vi "Requests.vi"(8 "error in (no error)":errorcluster, 9 "write enable":bool=TRUE, 11 "ICPCON ET7024 in":refnum<class "ICPCON ET-7024AO.lvclass">) -> (0 "error out":errorcluster, 3 "ICPCON ET7024 out":refnum<class "ICPCON ET-7024AO.lvclass">)   [LabVIEW 2021, in "ICPCON ET-7024AO.lvclass"]
uses:
  ICPCON ET-7024AO.lvclass
  D:/my_projects/projects/21/Master CR/Master CR.lvclass
  D:/my_projects/projects/21/Master CR/Devices/ET7000/TCP/TCP.lvclass
  Master CR.lvclass/Master CR.ctl
  Modbus_v121c/Modbus Data Unit/Modbus Data Unit.lvclass/Modbus Data Unit.ctl
  Modbus_v121c/Network Protocol/Network Master/Network Master.lvclass/Network Master.ctl
  Network Protocol/Read Network Protocol.vi
  Modbus_v121c/Master Function Definition/Write Multiple Registers Request.vi
  Modbus_v121c/Master Function Definition/Function data mismatch error.vi
  Modbus_v121c/Master Function Definition/Write Multiple Registers Response.vi
  Modbus_v121c/Network Protocol/Network Master/Read write Master.vi
  Modbus_v121c/Master Function Definition/Read Holding Registers Request.vi
  Modbus_v121c/Master Function Definition/Read Holding Registers Response.vi
  Modbus_v121c/Modbus Data Unit/Construct PDU.vi
  Modbus_v121c/Utility/U16s to Bytes.vi
  Modbus_v121c/Master Function Definition/Function code mismatch error.vi
  Modbus_v121c/Data Model/Error Generator.vi
  Modbus_v121c/Modbus Data Unit/Deconstruct PDU.vi
  Modbus_v121c/Utility/Bytes to U16s.vi
  TCP/TCP.lvclass
  Modbus_v121c/Network Protocol/Network Master/Network Master.lvclass
  Modbus_v121c/Modbus Data Unit/Modbus Data Unit.lvclass
  Modbus_v121c/Data Model/Device Data Model.lvclass
  Modbus_v121c/Transmission Data Unit/Transmission Data Unit.lvclass
  Master CR.lvclass
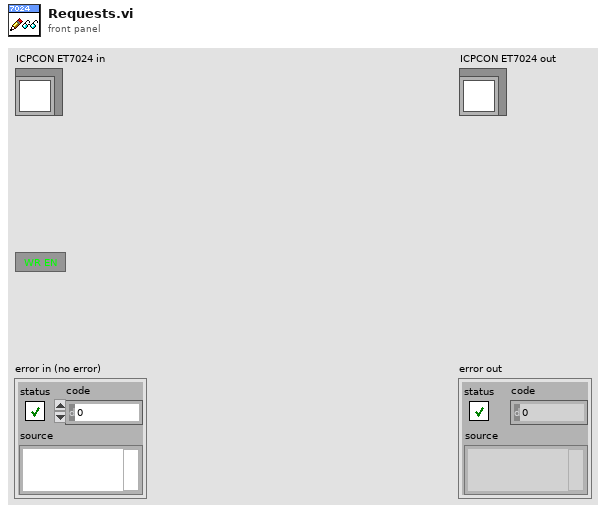
[diagram p1: front panel]
types:
  T1 = typedef "Device Data Model.lvclass/N channel.ctl" = cluster{"N DI channel":i32, "N DO channel":i32, "N AI channel":i32, "N AO channel":i32}
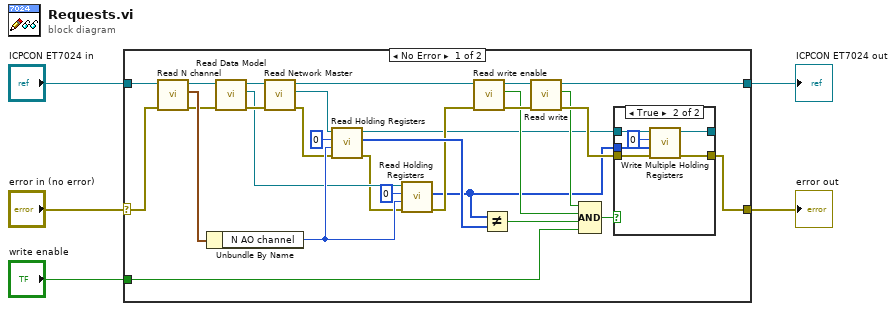
[diagram p0: block diagram]
diagram:
  n1 = case shown="No Error" "error in (no error)" {
    selector: "error in (no error)" -> [w31 w44]
    tunnel: [w27 w44] -> w3
    tunnel: [w26 w43] -> w4
    tunnel: "ICPCON ET7024 in" -> [w33 w43]
    tunnel: "write enable" -> [w28 _]
    frame No Error {
      n2 = call "Read N channel.vi"("error in (no error)"=w31, "Master CR in"=w33) -> ("error out"=w30:errorcluster, "N channel"=w34:T1, "Master CR out"=w32:refnum<class "ICPCON ET-7024AO.lvclass">)  [unwired: 7 in]
      n3 = Unbundle By Name(w34) -> ("N AO channel"=w29:i32)
      n4 = call "Read Data Model.vi"("error in (no error)"=w30, "Master CR in"=w32) -> ("error out"=w24:errorcluster, "Data Model"=w20:refnum<class "Device Data Model.lvclass">, "Master CR out"=w25:refnum<class "ICPCON ET-7024AO.lvclass">)  [unwired: 7 in]
      n5 = call "Read Network Master.vi"("error in (no error)"=w24, "TCP in"=w25) -> ("error out"=w21:errorcluster, "Network Master"=w22:refnum<class "Network Master.lvclass">, "TCP out"=w23:refnum<class "ICPCON ET-7024AO.lvclass">)  [unwired: 7 in]
      n6 = call "Read Holding Registers.vi"("error in (no error)"=w21, "number of holding registers"=w29, "starting address"=u16 0, "Modbus master in"=w22) -> ("error out"=w10:errorcluster, "register values"=w12:u16[], "Modbus master out"=w6:refnum<class "Network Master.lvclass">)  [unwired: 5 in]
      n7 = call-dynamic "Read Holding Registers.vi"("error in"=w10, "number of registers"=w29, "starting address"=u16 0, "device data model in"=w20) -> ("error out"=w11:errorcluster, "data"=w7:u16[])  [unwired: 5 in, 1 out]
      n8 = call "Read write enable.vi"("error in (no error)"=w11, "Master CR in"=w23) -> ("error out"=w16:errorcluster, "write enable"=w8:bool, "Master CR out"=w17:refnum<class "ICPCON ET-7024AO.lvclass">)  [unwired: 7 in]
      n9 = Not Equal?(x=w7, y=w12) -> (x != y?=w18:bool)
      n10 = call "Read write.vi"("error in (no error)"=w16, "Master CR in"=w17) -> ("error out"=w15:errorcluster, "Write"=w9:bool, "Master CR out"=w26:refnum<class "ICPCON ET-7024AO.lvclass">)  [unwired: 7 in]
      n11 = Compound Arithmetic op=AND(w9, w8, w18, w28) -> (w19:bool)
      n12 = case shown="True" w19 {
        tunnel: w15 -> [w36 w41]
        tunnel: [w36 w39] -> w27
        tunnel: w7 -> [_ w40]
        tunnel: [w35 w38] -> _
        tunnel: w6 -> [w35 w37]
        frame False {
        }
        frame True {
          n13 = call "Write Multiple Holding Registers.vi"("error in (no error)"=w41, "holding register values"=w40, "starting address"=u16 0, "Modbus master in"=w37) -> ("error out"=w39:errorcluster, "Modbus master out"=w38:refnum<class "Network Master.lvclass">)  [unwired: 6 in]
        }
      }
    }
    frame Error {
    }
  }
  "error out" <- w3
  "ICPCON ET7024 out" <- w4
